vi "Recursive Add Tag.vi"(8 "error in (no error)":errorcluster, 9 "Child Text":string[](array[string]), 10 "Tag":string, 11 "Tag Tree In":refnum<class "Tag Tree.lvclass">) -> (0 "error out":errorcluster, 3 "Tag Tree Out":refnum<class "Tag Tree.lvclass">)   [LabVIEW 2020, in "Tag Tree.lvclass"]
uses:
  Tag Tree.lvclass
  Tag Tree.lvclass/Tag Tree.ctl
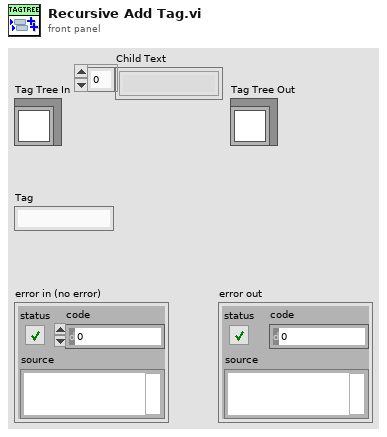
[diagram p1: front panel]
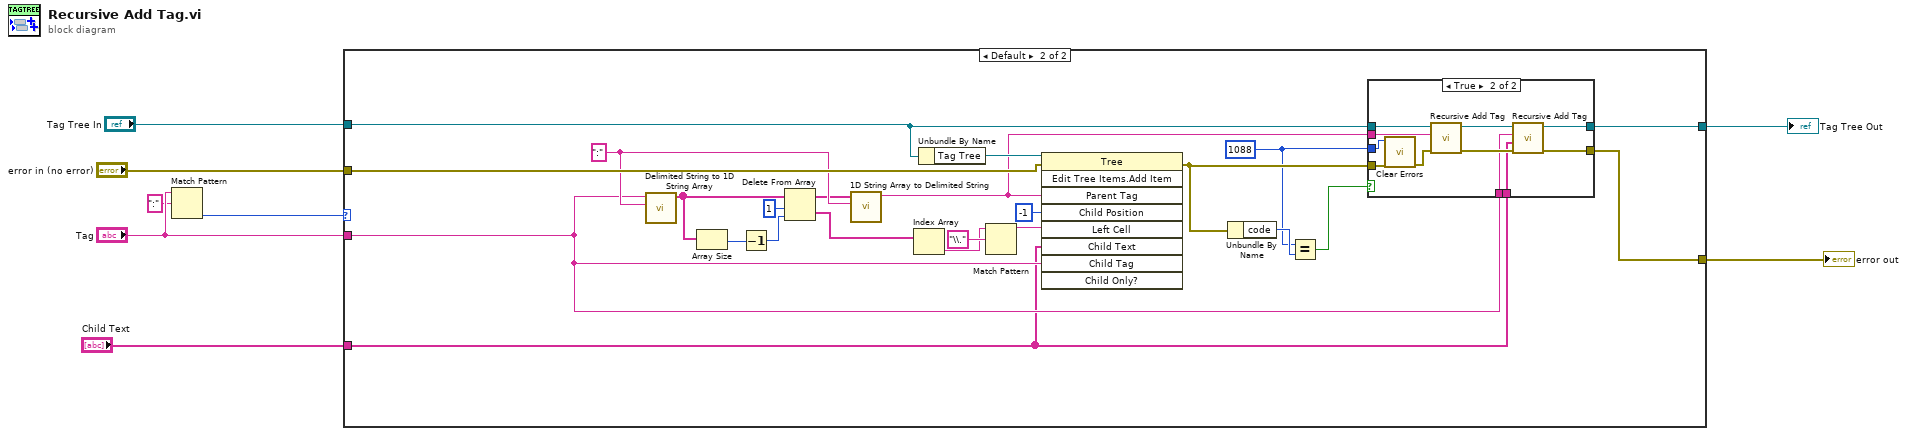
[diagram p0: block diagram]
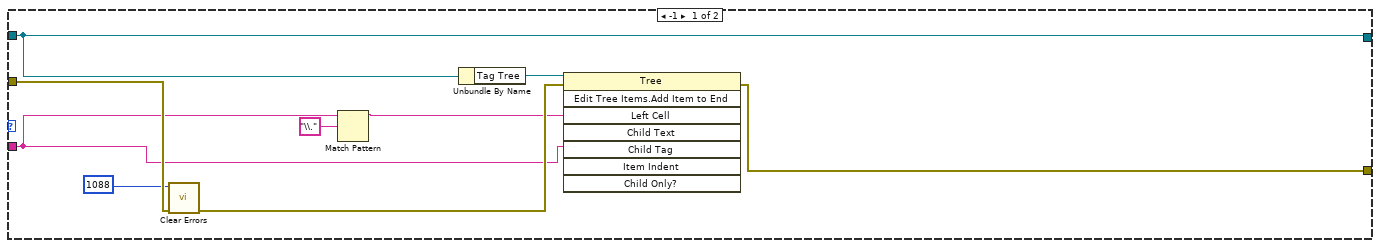
[diagram p2: hidden frame]
diagram:
  n1 = Match Pattern(string="Tag", regular expression=":") -> (offset past match=w2:i32)  [unwired: 1 in, 3 out]
  n2 = case shown="Default" w2 {
    tunnel: "error in (no error)" -> [w14 w40]
    tunnel: [w15 w29] -> w7
    tunnel: "Tag Tree In" -> [w16 w28]
    tunnel: [w16 w27] -> w5
    tunnel: "Tag" -> [w11 w24]
    tunnel: "Child Text" -> [_ w22]
    frame -1 {
      n3 = call <vilib>:"Clear Errors.vi"("error in (no error)"=w14, "specific error code to clear (0: all)"=1088) -> ("error out"=w12:errorcluster)  [unwired: 4 in, 1 out]
      n4 = Match Pattern(string=w11, regular expression="\\.") -> (before substring=w10:string)  [unwired: 1 in, 3 out]
      n5 = Unbundle By Name(w16) -> ("Tag Tree"=w17:refnum<vi>)
      n6 = invoke class="Tree" method="Edit Tree Items.Add Item to End"(reference=w17, error in=w12, "Left Cell"=w10, "Child Tag"=w11) -> (error out=w15:errorcluster)  [unwired: 4 in, 7 out]
    }
    frame Default {
      w21 = 1088
      w36 = ":" ("delimiter")
      n7 = call <vilib>:"Delimited String to 1D String Array.vi"("delimiter"=w36, "delimited string"=w24) -> ("string array"=w33:string[])  [unwired: 9 in]
      n8 = Array Size(array=w33) -> (size(s)=w31:i32)
      n9 = Decrement(x=w31) -> (x-1=w32:i32)
      n10 = Delete From Array(array=w33, length=1, index=w32) -> (deleted portion=w38:string[], array with subset deleted=w35:string[])
      n11 = call <vilib>:"1D String Array to Delimited String.vi"("delimiter"=w36, "string array"=w35) -> ("delimited string"=w26:string)  [unwired: 9 in]
      n12 = Index Array(array=w38) -> (element=w19:string)  [unwired: 1 in]
      n13 = Unbundle By Name(w28) -> ("Tag Tree"=w37:refnum<vi>)
      n14 = Match Pattern(string=w19, regular expression="\\.") -> (before substring=w18:string)  [unwired: 1 in, 3 out]
      n15 = invoke class="Tree" method="Edit Tree Items.Add Item"(reference=w37, error in=w40, "Parent Tag"=w26, "Child Position"=-1, "Left Cell"=w18, "Child Text"=w22, "Child Tag"=w24) -> (error out=w30:errorcluster)  [unwired: 2 in, 8 out]
      n16 = Unbundle By Name(w30) -> ("code"=w39:i32)
      n17 = Equal?(x=w21, y=w39) -> (x = y?=w25:bool)
      n18 = case shown="True" w25 {
        tunnel: w30 -> [w41 w45]
        tunnel: [w41 w48] -> w29
        tunnel: w28 -> [w42 w53]
        tunnel: [w42 w50] -> w27
        tunnel: w26 -> [_ w52]
        tunnel: w24 -> [_ w47]
        tunnel: w22 -> [_ w46]
        tunnel: w21 -> [_ w44]
        frame False {
        }
        frame True {
          n19 = call <vilib>:"Clear Errors.vi"("error in (no error)"=w45, "specific error code to clear (0: all)"=w44) -> ("error out"=w43:errorcluster)  [unwired: 4 in, 1 out]
          n20 = call "Recursive Add Tag.vi"("error in (no error)"=w43, "Tag"=w52, "Tag Tree In"=w53) -> ("error out"=w49:errorcluster, "Tag Tree Out"=w51:refnum<class "Tag Tree.lvclass">)  [unwired: 7 in]
          n21 = call "Recursive Add Tag.vi"("error in (no error)"=w49, "Child Text"=w46, "Tag"=w47, "Tag Tree In"=w51) -> ("error out"=w48:errorcluster, "Tag Tree Out"=w50:refnum<class "Tag Tree.lvclass">)  [unwired: 6 in]
        }
      }
    }
  }
  "error out" <- w7
  "Tag Tree Out" <- w5
